vi "PH_DeformableMirror.constructor.vi"(0 "name":string, 2 "data in":string, 5 "error in(no error)":errorcluster) -> (14 "i ref out":refnum<vi>, 16 "data out":string, 19 "error out":errorcluster)   [LabVIEW 2014, in "PH_DeformableMirror.lvlib"]
doc: "This is the constructor of the PH_DeformableMirror class. \n\nLicense Agreement for this software:\n\nCopyright (C)\nGesellschaft für Schwerionenforschung, GSI\nPlanckstr. 1\n64291 Darmstadt\nGermany\n\nContact: D.Beck@gsi.de \n\nThis program is free software; you can redistribute it and/or modify it under the terms of the \nGNU General Public License as published by the Free Software Foundation; either version 2 of \nthe license, or (at your option) any later version.\n\nThis program is distributed in the hope that it will be useful, but WITHOUT ANY WARRANTY; \nwithout even the implied warranty of MERCHANTABILITY or FITNESS FOR A PARTICULAR PURPOSE. See the GNU General License for more details (http://www.gnu.org).\n\nGesellschaft für Schwerionenforschung, GSI\nPlanckstr. 1, 64291 Darmstadt, Germany\nFor all questions and ideas contact: M.Richter@gsi.de, H.Brand@gsi.de or D.Beck@gsi.de.\nLast update: 16-JUN-2004"
uses:
  PH_DeformableMirror.lvlib
  PH_Basics/PH_Class/PH_Class.lvlib
  PH_Basics/PH_StatusHandler/PH_StatusHandler.lvlib
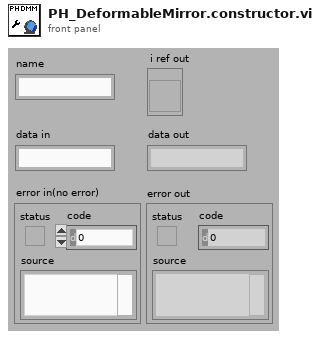
[diagram p1: front panel]
types:
  T1 = enum16{"SetAttribute", "GetAttribute", "CreateAttribute", "DestroyAttribute", "DestroyAllAtributes"}
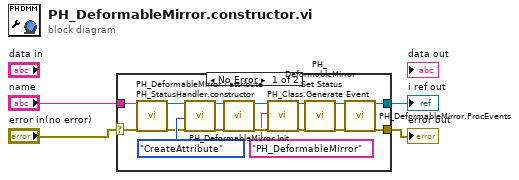
[diagram p0: block diagram]
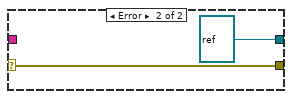
[diagram p2: hidden frame]
diagram:
  n1 = case shown="No Error" "error in(no error)" {
    selector: "error in(no error)" -> [w18 w22]
    tunnel: "name" -> [w14 _]
    tunnel: [w20 refnum<vi> refnum ("i ref out")] -> w3
    tunnel: [w19 w22] -> w2
    frame No Error {
      n2 = call "PH_StatusHandler.constructor.vi"("name"=w14, "error in(no error)"=w18) -> ("i ref out"=w6:refnum<vi>, "error out"=w5:errorcluster)  [unwired: 15 in, 1 out]
      n3 = call "PH_DeformableMirror.i attribute.vi"("VI Refnum"=w6, "Action"=T1."CreateAttribute", "error in (no error)"=w5) -> ("VI Refnum out"=w8:refnum<vi>, "error out"=w7:errorcluster)  [unwired: 14 in, 1 out]
      n4 = call "PH_DeformableMirror.Init.vi"("VI in"=w8, "error in (no error)"=w7) -> ("VI out"=w10:refnum<vi>, "error out"=w11:errorcluster)  [unwired: 16 in]
      n5 = call "PH_Class.Generate Event.vi"("i ref in"=w10, "Class"="PH_DeformableMirror", "error in (no error)"=w11) -> ("i ref out"=w15:refnum<vi>, "error out"=w16:errorcluster)  [unwired: 15 in]
      n6 = call "PH_DeformableMirror.Set Status.vi"("i ref in"=w15, "error in"=w16) -> ("i ref out"=w13:refnum<vi>, "error out"=w12:errorcluster)  [unwired: 16 in]
      n7 = call "PH_DeformableMirror.ProcEvents.vi"("i ref in"=w13, "error in"=w12) -> ("i ref out"=w20:refnum<vi>, "error out"=w19:errorcluster)  [unwired: 16 in]
    }
    frame Error {
    }
  }
  "i ref out" <- w3
  "error out" <- w2
